vi "Update Channels.vi"(8 "error in (no error)":errorcluster, 9 "Analog":bool, 10 "Previous Number of Channels":i32=8, 11 "Output Sequencer in":refnum<class "Output Sequencer.lvclass">) -> (0 "error out":errorcluster, 1 "Channels to Remove":string[](array[string]), 3 "Output Sequencer out":refnum<class "Output Sequencer.lvclass">, 5 "Channels to Add":refnum<class "Producer Channel.lvclass">[](array[class]))   [LabVIEW 2020, in "Output Sequencer.lvlib" / "Output Sequencer.lvclass"]
uses:
  Output Sequencer.lvclass
  <vilib>/FlexLogger/SDK/PluginSDK.lvlibp/PEFClasses/SDK/Producer Channel/Producer Channel.lvclass
  Output Sequencer.lvclass/Output Sequencer.ctl
  <vilib>/FlexLogger/SDK/PluginSDK.lvlibp/PEFClasses/SDK/Channel/Data Type_v2.ctl
  Globals/Global Strings.vi
  <vilib>/FlexLogger/SDK/PluginSDK.lvlibp/PEFClasses/SDK/Producer Channel/Create Producer Channel_v2.vi
  <vilib>/FlexLogger/SDK/PluginSDK.lvlibp/PEFClasses/SDK/Plugin/Plugin.lvclass
  <vilib>/FlexLogger/SDK/PluginSDK.lvlibp
  <vilib>/FlexLogger/SDK/PluginSDK.lvlibp/PEFClasses/SDK/Channel/Channel.lvclass
  C:/Program Files/National Instruments/LabVIEW 2024/vi.lib/FlexLogger/SDK/PluginSDK.lvlibp/PEFClasses/SDK/Plugin/Plugin.lvclass
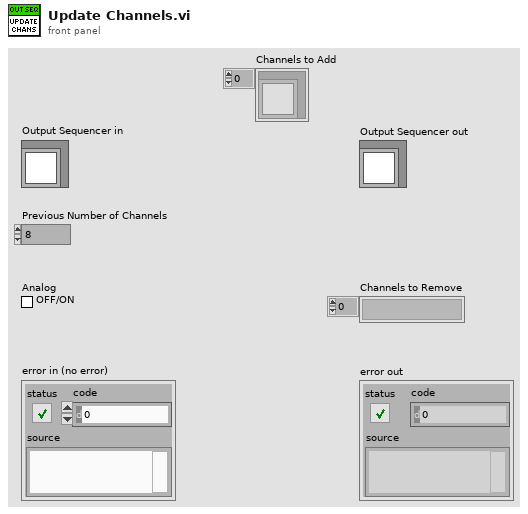
[diagram p1: front panel]
types:
  T1 = typedef "PluginSDK.lvlibp/Channel.lvclass/Data Type_v2.ctl" = u16
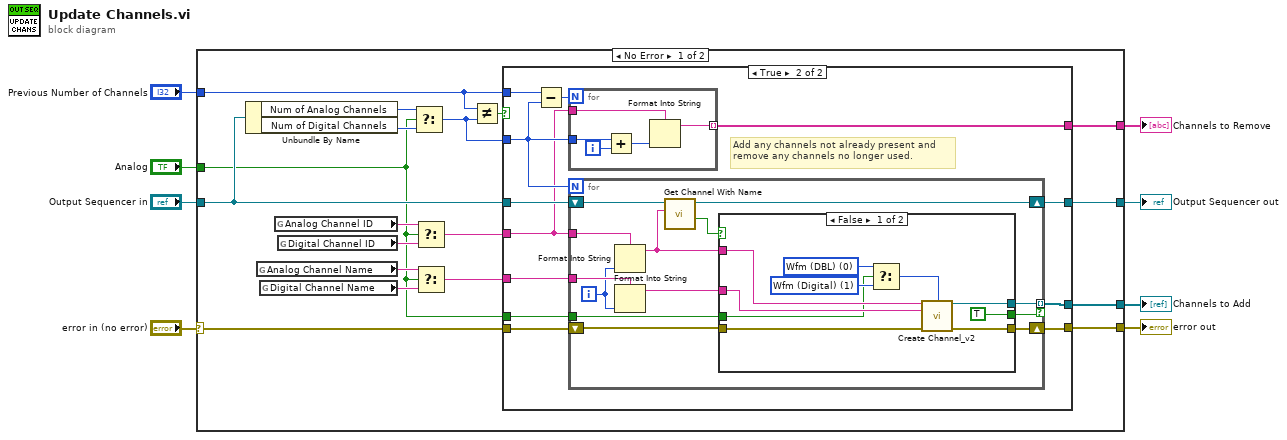
[diagram p0: block diagram]
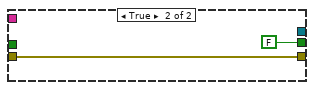
[diagram p3: hidden frame]
diagram:
  n1 = case shown="No Error" "error in (no error)" {
    selector: "error in (no error)" -> [w9 w70]
    tunnel: [w22 w71] -> w8
    tunnel: [w21 w70] -> w7
    tunnel: [w20 _] -> w6
    tunnel: [w19 _] -> w5
    tunnel: "Output Sequencer in" -> [w15 w71]
    tunnel: "Analog" -> [w12 _]
    tunnel: "Previous Number of Channels" -> [w11 _]
    frame No Error {
      n2 = Unbundle By Name(w15) -> ("Num of Analog Channels"=w14:i32, "Num of Digital Channels"=w13:i32)
      n3 = global read "Global Strings.vi" "Analog Channel Name"() -> (w17:string)
      n4 = global read "Global Strings.vi" "Digital Channel Name"() -> (w18:string)
      n5 = global read "Global Strings.vi" "Analog Channel ID"() -> (w25:string)
      n6 = global read "Global Strings.vi" "Digital Channel ID"() -> (w24:string)
      n7 = Select(t=w14, s=w12, f=w13) -> (s? t:f=w10:i32)
      n8 = Select(t=w25, s=w12, f=w24) -> (s? t:f=w23:string)
      n9 = Select(t=w17, s=w12, f=w18) -> (s? t:f=w16:string)
      n10 = Not Equal?(x=w11, y=w10) -> (x != y?=w26:bool)
      n11 = case shown="True" w26 {
        tunnel: w11 -> [_ w39]
        tunnel: w10 -> [_ w36]
        tunnel: w15 -> [w28 w32]
        tunnel: w9 -> [w27 w31]
        tunnel: [w28 w32] -> w22
        tunnel: [w27 w34] -> w21
        tunnel: w23 -> [_ w30]
        tunnel: w12 -> [_ w37]
        tunnel: [_ w35] -> w20
        tunnel: [_ w33] -> w19
        tunnel: w16 -> [_ w29]
        frame False {
        }
        frame True {
          # "Add any channels not already present and\nremove any channels no longer used."
          n12 = Subtract(x=w39, y=w36) -> (x-y=w38:i32)
          n13 = for {
            N: w38 -> [_]
            tunnel: [w65] -> w35 mode=indexing
            tunnel: w36 -> [w68]
            tunnel: w30 -> [w66]
            i -> [w69]
            n14 = Add(x=w68, y=w69) -> (x+y=w67:i32)
            n15 = Format Into String(format string=w66, w67) -> (resulting string=w65:string)  [unwired: 2 in, 1 out]
          }
          n16 = for {
            N: w36 -> [_]
            tunnel: [w51] -> w33 mode=indexing if=w46
            shift-right: [w50] -> w34
            shift-left: w31 -> [w49]
            tunnel: w30 -> [w48]
            tunnel: w37 -> [w47]
            tunnel: w29 -> [w43]
            shift-right: [w40] -> _
            shift-left: w32 -> [w52]
            i -> [w41]
            n17 = Format Into String(format string=w48, w41) -> (resulting string=w45:string)  [unwired: 2 in, 1 out]
            n18 = Format Into String(format string=w43, w41) -> (resulting string=w42:string)  [unwired: 2 in, 1 out]
            n19 = call <vilib>:"Get Channel With Name.vi"("Name"=w45, "Plugin in"=w52) -> ("Found?"=w44:bool, "Plugin out"=w40:refnum<class "Output Sequencer.lvclass">)  [unwired: 7 in, 1 out]
            n20 = case shown="False" w44 {
              tunnel: w45 -> [w61 _]
              tunnel: [w59 _] -> w51
              tunnel: [TRUE FALSE] -> w46
              tunnel: [w57 w64] -> w50
              tunnel: w49 -> [w58 w64]
              tunnel: w47 -> [w54 _]
              tunnel: w42 -> [w60 _]
              frame False {
                w55 = T1 1 items=["Wfm (DBL)", "Wfm (Digital)", "String"] ("Data Type")
                w56 = T1 0 items=["Wfm (DBL)", "Wfm (Digital)", "String"] ("Data Type")
                n21 = Select(t=w56, s=w54, f=w55) -> (s? t:f=w53:T1)
                n22 = call-poly <vilib>:"Create Channel_v2.vi"("Unique Channel Identifier"=w61, "Data Type"=w53, "Default Channel Name"=w60, "error in (no error)"=w58) -> ("Producer Channel"=w59:refnum<class "Producer Channel.lvclass">, "error out"=w57:errorcluster)  [unwired: 10 in]
              }
              frame True {
              }
            }
          }
        }
      }
    }
    frame Error {
    }
  }
  "Output Sequencer out" <- w8
  "error out" <- w7
  "Channels to Remove" <- w6
  "Channels to Add" <- w5
